vi "osie na grafie jazda.vi"(4 "Y axis rotation":i32, 6 "X axis rotation":i32, 8 "Y axis":i32, 9 "X axis":i32) -> (5 "graph 1":cluster{i32[], i32[]}[](graph))   [LabVIEW 2015]
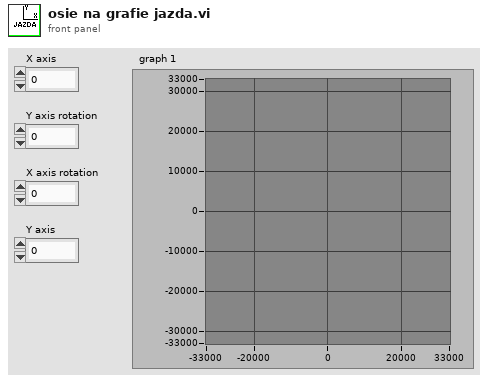
[diagram p1: front panel]
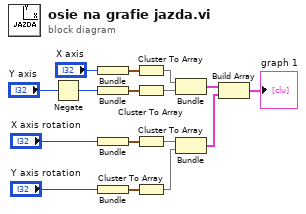
[diagram p0: block diagram]
diagram:
  n1 = Negate(x="Y axis") -> (-x=w4:i32)
  n2 = Bundle("X axis"="X axis") -> (w3:cluster{"X axis":i32})  [unwired: 1 in]
  n3 = Bundle(w4) -> (w7:cluster{i32})  [unwired: 1 in]
  n4 = Bundle("X axis rotation"="X axis rotation") -> (w9:cluster{"X axis rotation":i32})  [unwired: 1 in]
  n5 = Bundle("Y axis rotation"="Y axis rotation") -> (w8:cluster{"Y axis rotation":i32})  [unwired: 1 in]
  n6 = Cluster To Array(cluster=w3) -> (array=w2:i32[])
  n7 = Cluster To Array(cluster=w7) -> (array=w1:i32[])
  n8 = Cluster To Array(cluster=w9) -> (array=w11:i32[])
  n9 = Cluster To Array(cluster=w8) -> (array=w10:i32[])
  n10 = Bundle(w2, w1) -> (w15:cluster{i32[], i32[]})  [unwired: 1 in]
  n11 = Bundle(w11, w10) -> (w14:cluster{i32[], i32[]})  [unwired: 1 in]
  n12 = Build Array(w15, w14) -> (→"graph 1":cluster{i32[], i32[]}[])
